vi "dequeue.vi"(8 "error in (no error)":errorcluster, 11 "ComicVine_manager in":refnum<class "ComicVine_manager.lvclass">) -> (0 "error out":errorcluster, 1 "data":variant, 2 "cmd":T1, 3 "ComicVine_manager out":refnum<class "ComicVine_manager.lvclass">)   [LabVIEW 2024, in "ComicVine_manager.lvclass"]
uses:
  ComicVine_manager.lvclass
  ComicVine_manager.lvclass/ComicVine_manager.ctl
  states--enum.ctl
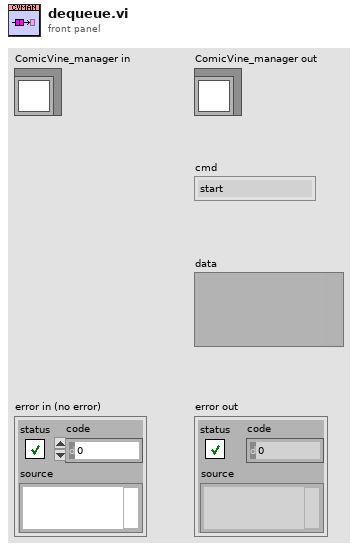
[diagram p1: front panel]
types:
  T1 = typedef "ComicVine_manager.lvclass/states--enum.ctl" = enum16{"start", "running", "shutdown"}
  T2 = typedef "ComicVine_manager.lvclass/queue.message--cluster.ctl" = cluster{"cmd":T1, "data":variant}
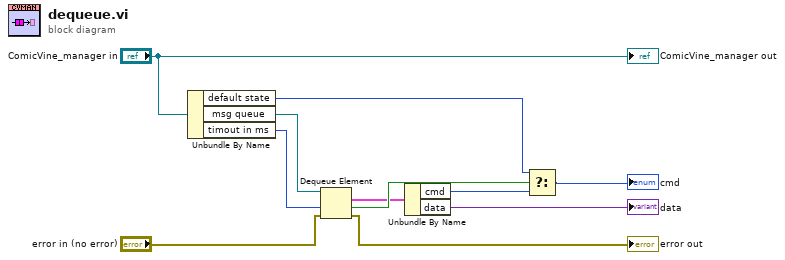
[diagram p0: block diagram]
diagram:
  n1 = Unbundle By Name("ComicVine_manager in") -> ("default state"=w6:T1, "msg queue"=w10:refnum<queue>, "timout in ms"=w11:i32)
  n2 = Dequeue Element(queue=w10, timeout in ms (-1)=w11, error in (no error)="error in (no error)") -> (element=w8:T2, timed out?=w9:bool, error out=→"error out":errorcluster)  [unwired: 1 out]
  n3 = Unbundle By Name(w8) -> ("cmd"=w7:T1, "data"=→"data":variant)
  n4 = Select(t=w6, s=w9, f=w7) -> (s? t:f=→"cmd":T1)
  "ComicVine_manager out" <- "ComicVine_manager in"
